vi "_Convert ADC Voltage.vi"(10 "SPI Read Array":u8[](array[numeric]), 11 "Vref (3.3V)":dbl=3.3) -> (0 "L":u8 format="%.0x", 1 "H":u8 format="%.0x", 2 "12-bit ADC Code":u16 format="%.0x", 3 "Converted Voltage (V)":dbl)   [LabVIEW 2014]
doc: "<b>-------------------------------------------------------</b>\n** Author: Derek Murray\n** Created: 22/08/2016\n** LV Version: LabVIEW 2014 Home SP1 (14.0.1f3 32-bit)\n<b>-------------------------------------------------------</b>\n\nConverts the data bytes read back from the MCP3008 to an equivalent voltage. Also returns the 10-bit ADC code. The correct reference voltage must be entered to the VI (default 3.3V). \n\n<b>-------------------------------------------------------</b>\n** Copyright/License\nPermission is hereby granted, free of charge, to any person obtaining a copy of this software and associated documentation files (the \"Software\"), to deal in the Software without restriction, including without limitation the rights to use, copy, modify, merge, publish, distribute, sublicense, and/or sell copies of the Software, and to permit persons to whom the Software is furnished to do so, subject to the following conditions:\nThe above copyright notice and this permission notice shall be included in all copies or substantial portions of the Software.\nTHE SOFTWARE IS PROVIDED \"AS IS\", WITHOUT WARRANTY OF ANY KIND, EXPRESS OR IMPLIED, INCLUDING BUT NOT LIMITED TO THE WARRANTIES OF MERCHANTABILITY, FITNESS FOR A PARTICULAR PURPOSE AND NONINFRINGEMENT. IN NO EVENT SHALL THE AUTHORS OR COPYRIGHT HOLDERS BE LIABLE FOR ANY CLAIM, DAMAGES OR OTHER LIABILITY, WHETHER IN AN ACTION OF CONTRACT, TORT OR OTHERWISE, ARISING FROM, OUT OF OR IN CONNECTION WITH THE SOFTWARE OR THE USE OR OTHER DEALINGS IN THE SOFTWARE."
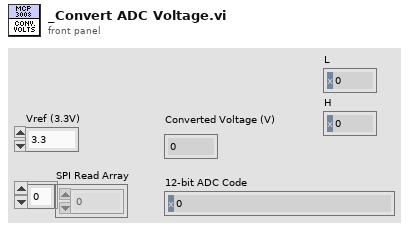
[diagram p1: front panel]
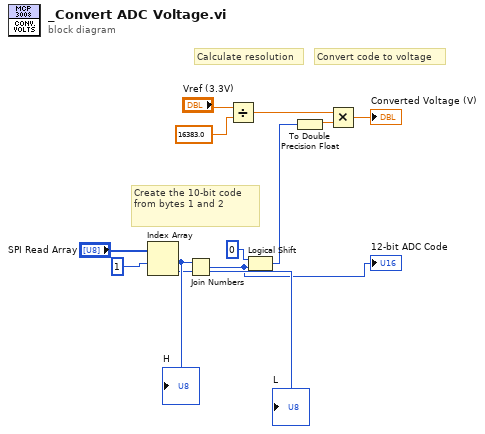
[diagram p0: block diagram]
diagram:
  # "Create the 10-bit code from bytes 1 and 2"
  # "Convert code to voltage"
  # "Calculate resolution"
  n1 = Index Array(array="SPI Read Array", index #1=1 ("index")) -> (element #1=w9:u8, element #2=w8:u8)  [unwired: 1 in]
  "L" <- w8
  "H" <- w9
  n2 = Join Numbers(hi=w9, lo=w8) -> ((hi.lo)=w1:u16)
  "12-bit ADC Code" <- w1
  n3 = Divide(x="Vref (3.3V)", y=16383.0) -> (x/y=w5:dbl)
  n4 = Logical Shift(y=i16 0, x=w1) -> (x << y=w3:u16)
  n5 = To Double Precision Float(number=w3) -> (double precision float=w4:dbl)
  n6 = Multiply(x=w5, y=w4) -> (x*y=→"Converted Voltage (V)":dbl)
